vi "SP SP - get subsubpanel.vi"(8 "error in (no error)":errorcluster, 10 "subpanel":string, 11 "subsubpanel":string) -> (0 "error out":errorcluster, 1 "references":T1, 2 "SubSubPanel found":bool, 3 "SubSubPanel VI":refnum<vi>)   [LabVIEW 2020, in "ui-testing.lvlib"]
uses:
  ui-testing.lvlib
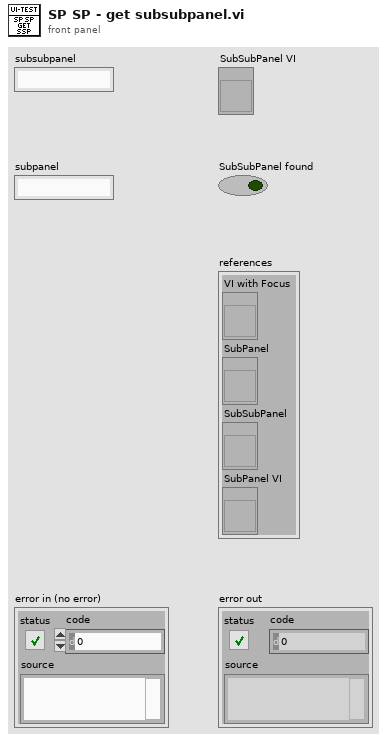
[diagram p1: front panel]
types:
  T1 = cluster{"VI with Focus":refnum<vi>, "SubPanel":refnum<vi>, "SubSubPanel":refnum<vi>, "SubPanel VI":refnum<vi>}
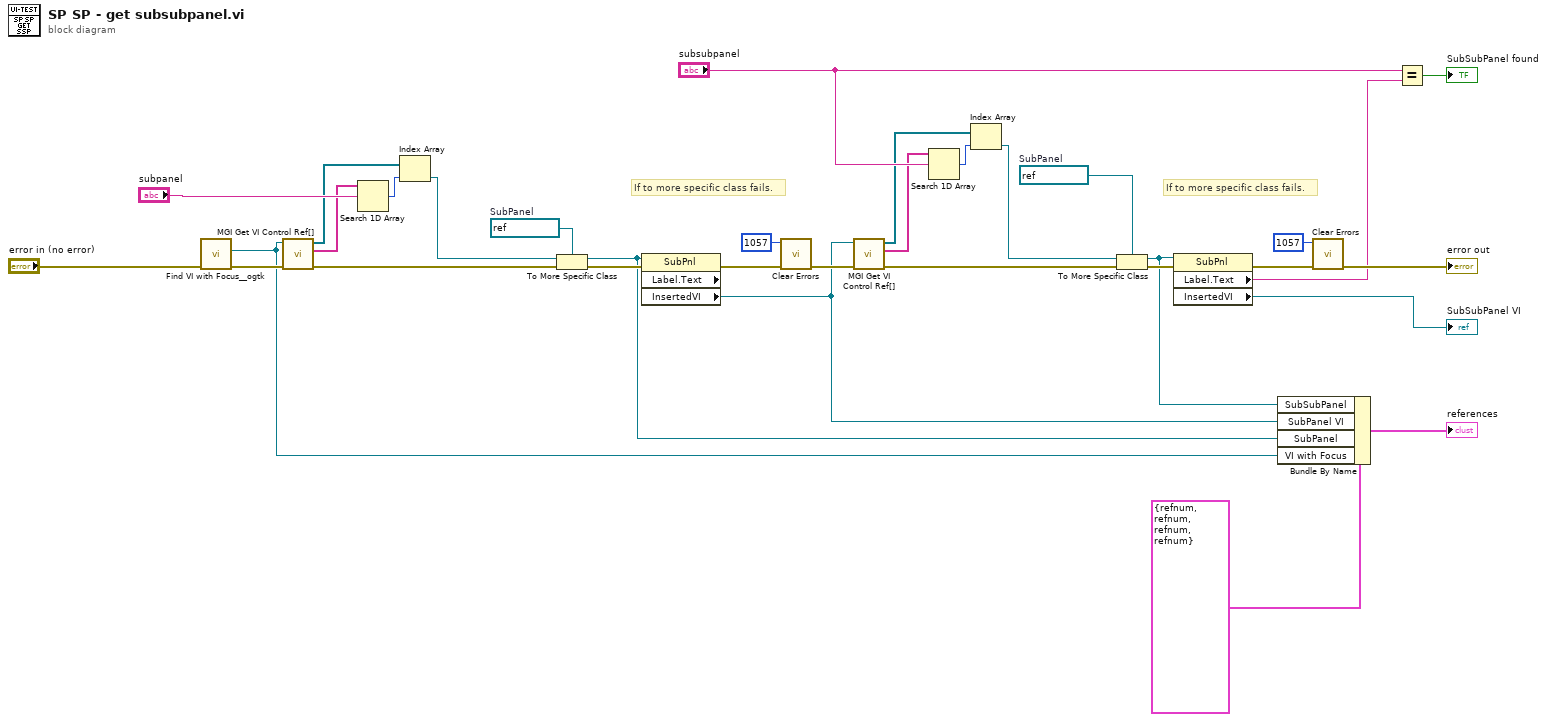
[diagram p0: block diagram]
diagram:
  w19 = refnum<vi> refnum  # SubPanel
  w16 = refnum<vi> refnum  # SubPanel
  # "If to more specific class fails."
  # "If to more specific class fails."
  n1 = call <userlib>:"Find VI with Focus__ogtk.vi"("error in"="error in (no error)") -> ("error out"=w11:errorcluster, "VI with Focus"=w5:refnum<vi>)  [unwired: 6 in, 3 out]
  n2 = call <userlib>:"MGI Get VI Control Ref[].vi"("error in"=w11, "VI (Caller)"=w5) -> ("error out"=w17:errorcluster, "Control Label Chain[i]"=w8:string[], "Control[i]"=w9:refnum<vi>[])  [unwired: 6 in, 1 out]
  n3 = Search 1D Array(1D array=w8, element="subpanel") -> (index of element=w10:i32)  [unwired: 1 in]
  n4 = Index Array(array=w9, index=w10) -> (element=w18:refnum<vi>)
  n5 = To More Specific Class(target class=w16, reference=w18, error in=w17) -> (specific class reference=w3:refnum<vi>, error out=w15:errorcluster)
  n6 = property class="SubPnl" props=["Label", "Text", "InsertedVI"](reference=w3, error in=w15) -> (error out=w13:errorcluster, "InsertedVI"=w2:refnum<vi>)  [unwired: 2 out]
  n7 = call <vilib>:"Clear Errors.vi"("error in (no error)"=w13, "specific error code to clear (0: all)"=1057) -> ("error out"=w30:errorcluster)  [unwired: 4 in, 1 out]
  n8 = call <userlib>:"MGI Get VI Control Ref[].vi"("error in"=w30, "VI (Caller)"=w2) -> ("error out"=w31:errorcluster, "Control Label Chain[i]"=w27:string[], "Control[i]"=w28:refnum<vi>[])  [unwired: 6 in, 1 out]
  n9 = Search 1D Array(1D array=w27, element="subsubpanel") -> (index of element=w29:i32)  [unwired: 1 in]
  n10 = Index Array(array=w28, index=w29) -> (element=w32:refnum<vi>)
  n11 = To More Specific Class(target class=w19, reference=w32, error in=w31) -> (specific class reference=w4:refnum<vi>, error out=w20:errorcluster)
  n12 = property class="SubPnl"(reference=w4, error in=w20) -> (error out=w24:errorcluster, "Label.Text"=w21:string, "InsertedVI"=→"SubSubPanel VI":refnum<vi>)  [unwired: 1 out]
  n13 = Bundle By Name(cluster=T1 {"VI with Focus"=refnum, "SubPanel"=refnum, "SubSubPanel"=refnum, "SubPanel VI"=refnum}, "SubSubPanel"=w4, "SubPanel VI"=w2, "SubPanel"=w3, "VI with Focus"=w5) -> (→"references":T1)
  n14 = call <vilib>:"Clear Errors.vi"("error in (no error)"=w24, "specific error code to clear (0: all)"=1057) -> ("error out"=→"error out":errorcluster)  [unwired: 4 in, 1 out]
  n15 = Equal?(x="subsubpanel", y=w21) -> (x = y?=→"SubSubPanel found":bool)
